vi "TCP-IP Mgr.Listener with Abort.vi"(8 "error in":errorcluster, 9 "Q.Abort":refnum<queue>, 11 "port":u16) -> (0 "error out":errorcluster, 1 "Aborted":bool, 2 "Connected":bool, 3 "Connection ID":refnum<k5>, 5 "remote address":string, 7 "remote port":u16)   [LabVIEW 2024, in "EQMF.lvlib" / "TCP-IP.lvlib"]
uses:
  TCP-IP.lvlib
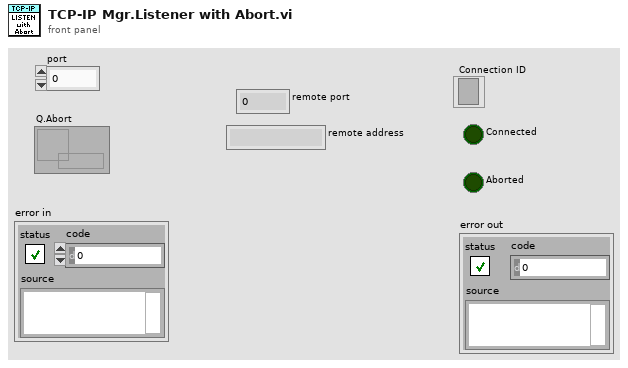
[diagram p1: front panel]
types:
  T1 = cluster{"Q.Abort":refnum<queue>, "listener ID":refnum<k5>, "Aborted":bool, "Connected":bool, "Error":errorcluster}
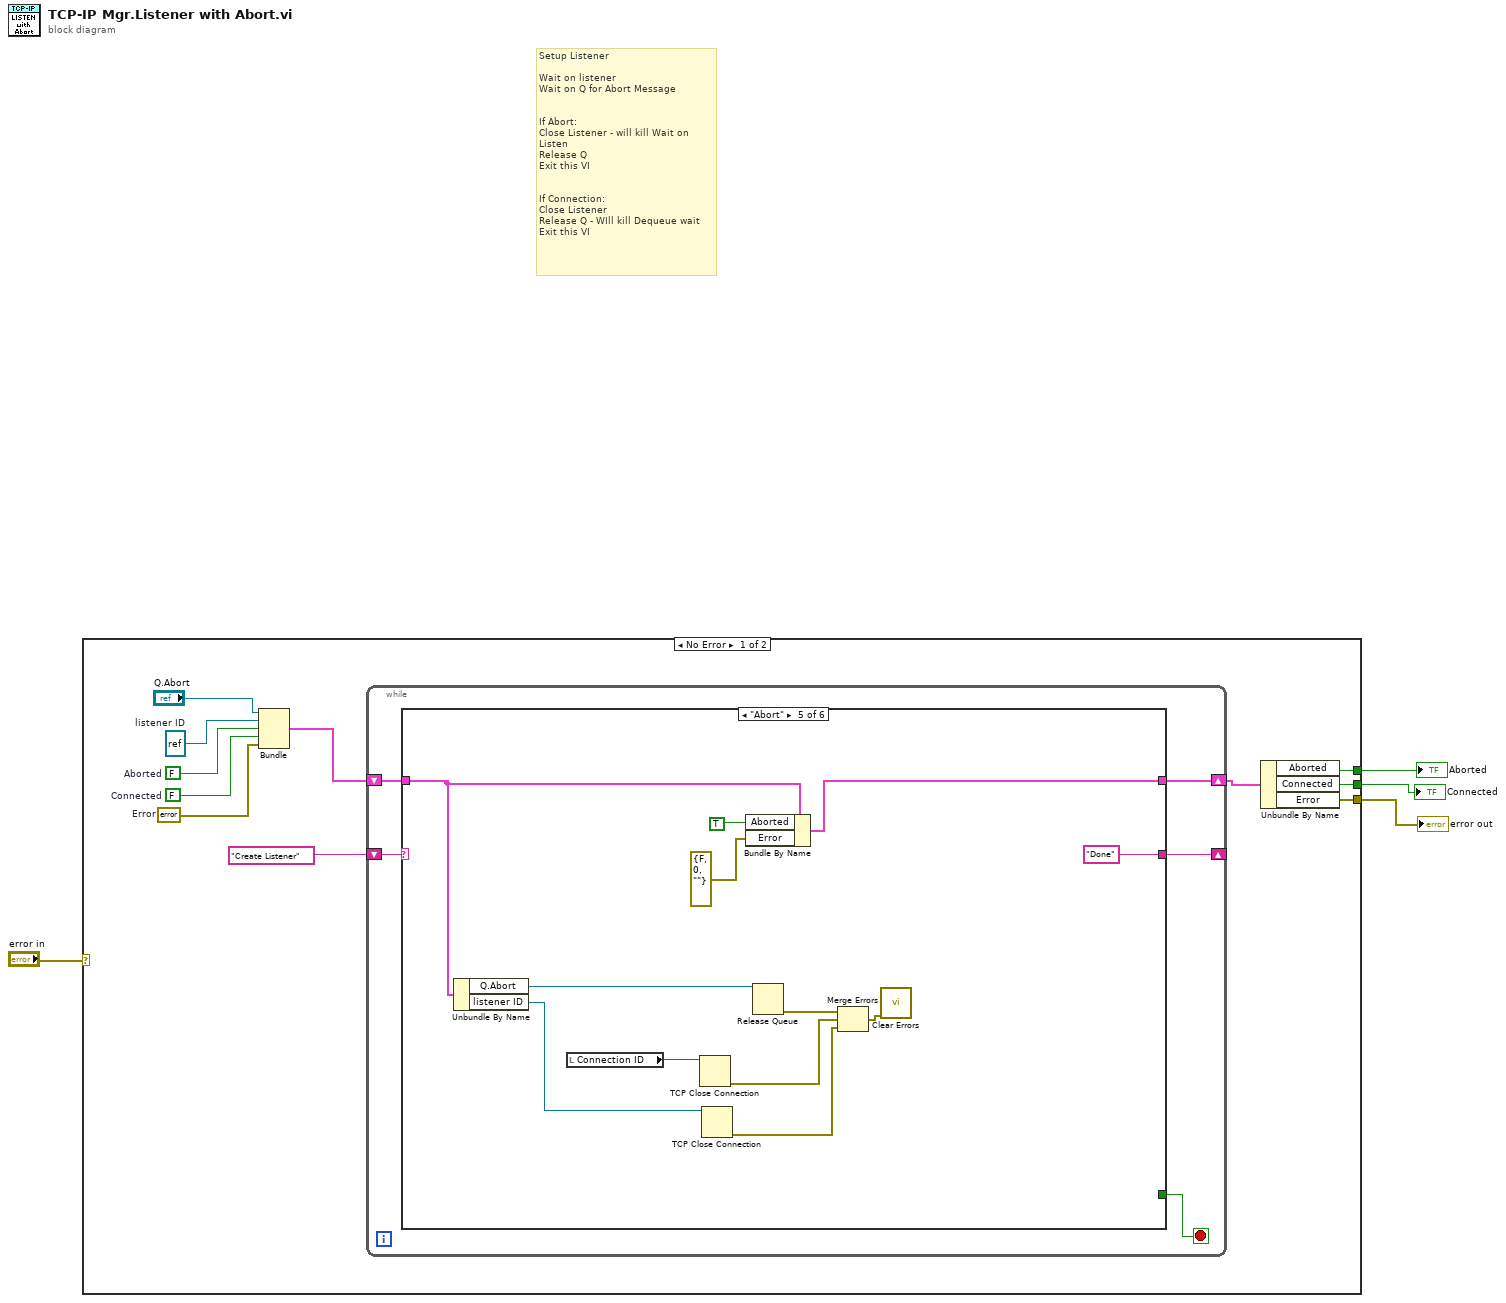
[diagram p0: block diagram]
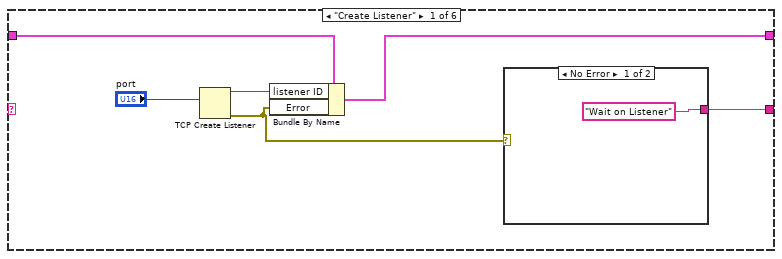
[diagram p2: hidden frame]
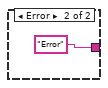
[diagram p3: hidden frame]
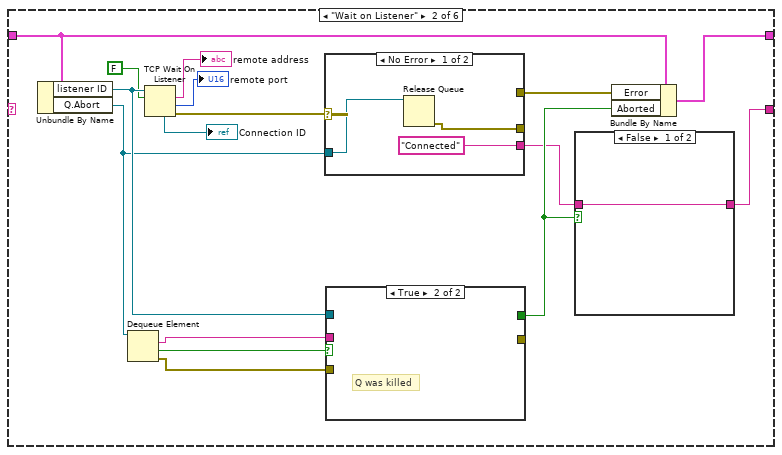
[diagram p4: hidden frame]
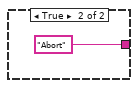
[diagram p5: hidden frame]
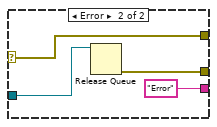
[diagram p6: hidden frame]
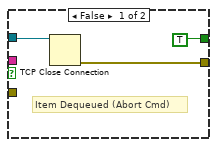
[diagram p7: hidden frame]
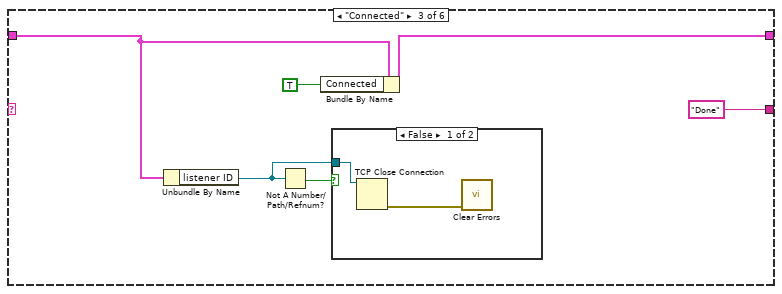
[diagram p8: hidden frame]
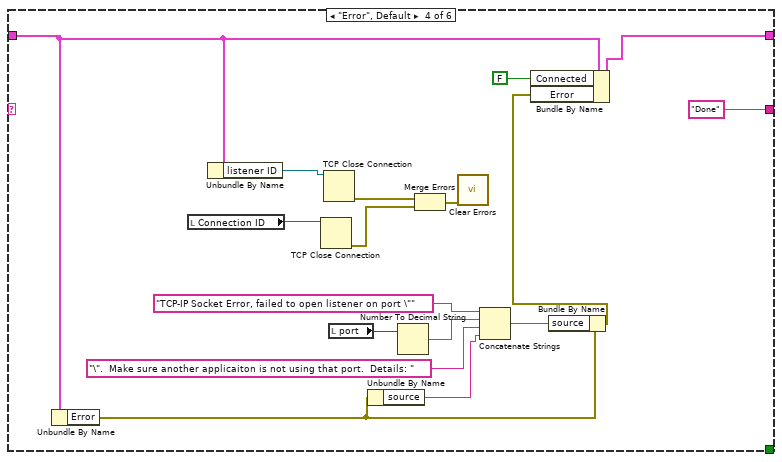
[diagram p10: hidden frame]
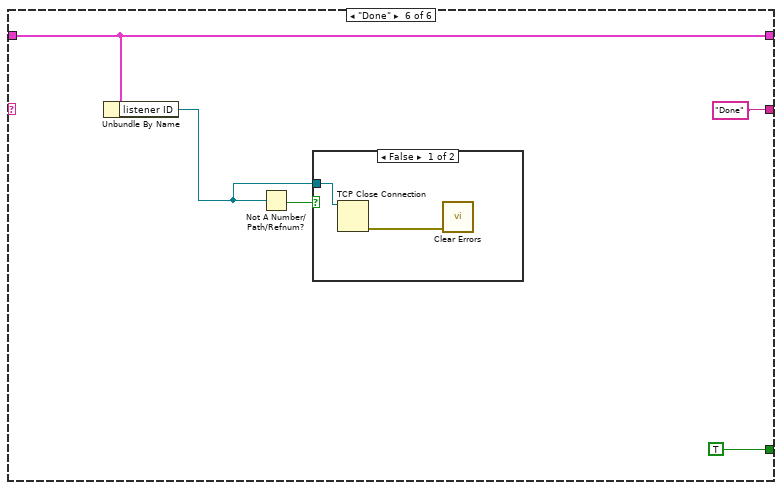
[diagram p11: hidden frame]
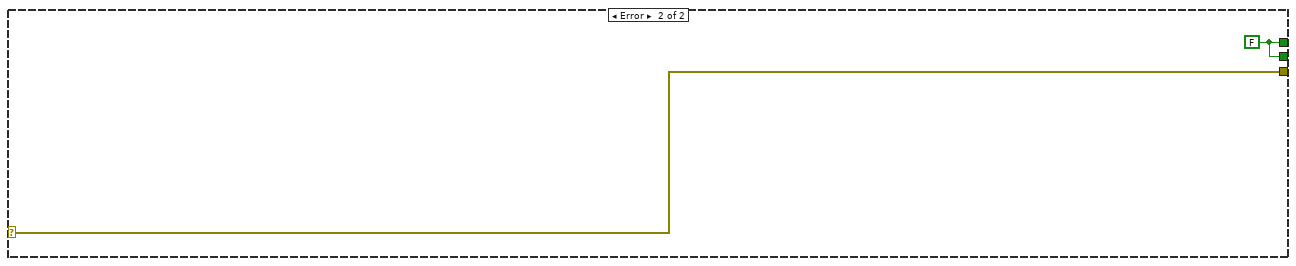
[diagram p13: hidden frame]
diagram:
  # "Setup Listener\n\nWait on listener\nWait on Q for Abort Message\n\n\nIf Abort:\nClose Listener - will kill Wait on Listen\nRelease Q\nExit this VI\n\n\nIf Connection:\nClose Listener\nRelease Q - WIll kill Dequeue wait\nExit this VI"
  n1 = case shown="No Error" "error in" {
    selector: "error in" -> [_ w102]
    tunnel: [w7 w101] -> w4
    tunnel: [w6 w101] -> w3
    tunnel: [w5 w102] -> w2
    frame No Error {
      w9 = FALSE  # Connected
      w10 = errorcluster {"status"=FALSE, "code"=0, "source"=""}  # Error
      w11 = FALSE  # Aborted
      w13 = refnum<k5> refnum  # listener ID
      n2 = Bundle("Q.Abort"="Q.Abort", "listener ID"=w13, "Aborted"=w11, "Connected"=w9, "Error"=w10) -> (w15:T1)  [unwired: 1 in]
      n3 = while {
        shift-right: [w17] -> _
        shift-left: "Create Listener" -> [w20]
        shift-right: [w18] -> w8
        shift-left: w15 -> [w19]
        stop <- w16 stop-if-true
        n4 = case shown="\"Abort\"" w20 {
          tunnel: w19 -> [w24 w37 w59 w72 w89 w96]
          tunnel: [w23 w36 w61 w80 w92 w96] -> w18
          tunnel: [w22 w34 "Done" "Done" "Done" "Done"] -> w17
          tunnel: [_ _ _ _ _ TRUE] -> w16
          frame "Create Listener" {
            n5 = TCP Create Listener(10:"port") -> (0:w21:errorcluster, 3:w25:refnum<k5>)  [unwired: 1 in, 4 out]
            n6 = Bundle By Name(cluster=w24, "listener ID"=w25, "Error"=w21) -> (w23:T1)
            n7 = case shown="No Error" w21 {
              tunnel: ["Wait on Listener" "Error"] -> w22
              frame No Error {
              }
              frame Error {
              }
            }
          }
          frame "Wait on Listener" {
            n8 = Unbundle By Name(w37) -> ("listener ID"=w40:refnum<k5>, "Q.Abort"=w38:refnum<queue>)
            n9 = Dequeue Element(queue=w38) -> (element=w30:string, timed out?=w41:bool, error out=w31:errorcluster)  [unwired: 2 in, 1 out]
            n10 = TCP Wait On Listener(10:FALSE, 11:w40) -> (0:w39:errorcluster, 1:→"remote port":u16, 2:→"remote address":string, 4:→"Connection ID":refnum<k5>)  [unwired: 1 in, 2 out]
            n11 = case shown="No Error" w39 {
              selector: w39 -> [_ w52]
              tunnel: w38 -> [w49 w51]
              tunnel: ["Connected" "Error"] -> w33
              tunnel: [_ w52] -> w32
              tunnel: [w47 w50] -> _
              frame No Error {
                n12 = Release Queue(queue=w49) -> (error out=w47:errorcluster)  [unwired: 2 in, 2 out]
              }
              frame Error {
                n13 = Release Queue(queue=w51) -> (error out=w50:errorcluster)  [unwired: 2 in, 2 out]
              }
            }
            n14 = case shown="True" w41 {
              tunnel: w40 -> [w55 _]
              tunnel: [TRUE _] -> w35
              tunnel: w31 -> [_ _]
              tunnel: [w54 _] -> _
              tunnel: w30 -> [_ _]
              frame False {
                # "Item Dequeued (Abort Cmd)"
                n15 = TCP Close Connection(connection ID=w55) -> (error out=w54:errorcluster)  [unwired: 2 in, 1 out]
              }
              frame True {
                # "Q was killed"
              }
            }
            n16 = case shown="False" w35 {
              tunnel: [w45 "Abort"] -> w34
              tunnel: w33 -> [w45 _]
              frame False {
              }
              frame True {
              }
            }
            n17 = Bundle By Name(cluster=w37, "Error"=w32, "Aborted"=w35) -> (w36:T1)
          }
          frame "Connected" {
            n18 = Unbundle By Name(w59) -> ("listener ID"=w57:refnum<k5>)
            n19 = Not A Number/Path/Refnum?(number/path/refnum=w57) -> (NaN/Path/Refnum?=w58:bool)
            n20 = Bundle By Name(cluster=w59, "Connected"=TRUE) -> (w61:T1)
            n21 = case shown="False" w58 {
              tunnel: w57 -> [w63 _]
              frame False {
                n22 = TCP Close Connection(connection ID=w63) -> (error out=w64:errorcluster)  [unwired: 2 in, 1 out]
                n23 = call <vilib>:"Clear Errors.vi"("error in (no error)"=w64) -> ()  [unwired: 5 in, 2 out]
              }
              frame True {
              }
            }
          }
          frame "Error", Default {
            n24 = Unbundle By Name(w72) -> ("Error"=w69:errorcluster)
            n25 = local read "Connection ID"() -> (w77:refnum<k5>)
            n26 = Unbundle By Name(w72) -> ("listener ID"=w78:refnum<k5>)
            n27 = TCP Close Connection(connection ID=w77) -> (error out=w66:errorcluster)  [unwired: 2 in, 1 out]
            n28 = TCP Close Connection(connection ID=w78) -> (error out=w67:errorcluster)  [unwired: 2 in, 1 out]
            n29 = local read "port"() -> (w76:u16)
            n30 = Unbundle By Name(w69) -> ("source"=w68:string)
            n31 = Number To Decimal String(number=w76) -> (decimal integer string=w75:string)  [unwired: 1 in]
            n32 = Merge Errors(w67, w66) -> (w65:errorcluster)
            n33 = call <vilib>:"Clear Errors.vi"("error in (no error)"=w65) -> ()  [unwired: 5 in, 2 out]
            n34 = Concatenate Strings("TCP-IP Socket Error, failed to open listener on port \"", w75, "\".  Make sure another applicaiton is not using that port.  Details: ", w68) -> (w70:string)
            n35 = Bundle By Name(cluster=w69, "source"=w70) -> (w71:errorcluster)
            n36 = Bundle By Name(cluster=w72, "Connected"=FALSE, "Error"=w71) -> (w80:T1)
          }
          frame "Abort" {
            n37 = Unbundle By Name(w89) -> ("Q.Abort"=w88:refnum<queue>, "listener ID"=w83:refnum<k5>)
            n38 = local read "Connection ID"() -> (w87:refnum<k5>)
            n39 = TCP Close Connection(connection ID=w87) -> (error out=w84:errorcluster)  [unwired: 2 in, 1 out]
            n40 = TCP Close Connection(connection ID=w83) -> (error out=w82:errorcluster)  [unwired: 2 in, 1 out]
            n41 = Bundle By Name(cluster=w89, "Aborted"=TRUE, "Error"=errorcluster {"status"=FALSE, "code"=0, "source"=""}) -> (w92:T1)
            n42 = Release Queue(queue=w88) -> (error out=w85:errorcluster)  [unwired: 2 in, 2 out]
            n43 = Merge Errors(w85, w84, w82) -> (w86:errorcluster)
            n44 = call <vilib>:"Clear Errors.vi"("error in (no error)"=w86) -> ()  [unwired: 5 in, 2 out]
          }
          frame "Done" {
            n45 = Unbundle By Name(w96) -> ("listener ID"=w94:refnum<k5>)
            n46 = Not A Number/Path/Refnum?(number/path/refnum=w94) -> (NaN/Path/Refnum?=w95:bool)
            n47 = case shown="False" w95 {
              tunnel: w94 -> [w99 _]
              frame False {
                n48 = TCP Close Connection(connection ID=w99) -> (error out=w100:errorcluster)  [unwired: 2 in, 1 out]
                n49 = call <vilib>:"Clear Errors.vi"("error in (no error)"=w100) -> ()  [unwired: 5 in, 2 out]
              }
              frame True {
              }
            }
          }
        }
      }
      n50 = Unbundle By Name(w8) -> ("Aborted"=w7:bool, "Connected"=w6:bool, "Error"=w5:errorcluster)
    }
    frame Error {
      w101 = FALSE
    }
  }
  "error out" <- w2
  "Aborted" <- w4
  "Connected" <- w3
